vi "Network - Send Start Session.vi"(8 "error in":errorcluster, 9 "Info":string, 10 "URL":string="127.0.0.1", 11 "Numeric":dbl) -> (0 "error out":errorcluster)   [LabVIEW 2010, in "Core SubVIs.lvlib"]
uses:
  Core SubVIs.lvlib
panel:
  out "Connected":bool
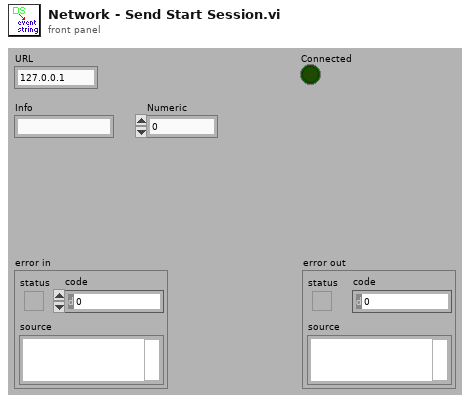
[diagram p1: front panel]
types:
  T1 = enum16{"Read", "Write", "ReadWrite", "BufferedRead", "BufferedReadWrite"}
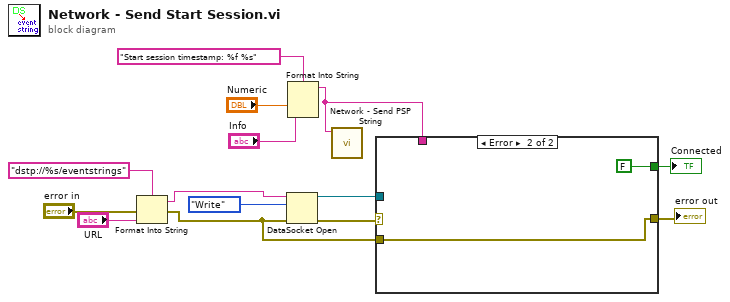
[diagram p0: block diagram]
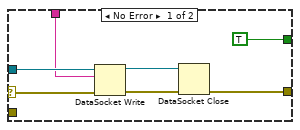
[diagram p2: hidden frame]
diagram:
  n1 = Format Into String(format string="dstp://%s/eventstrings", error in="error in", "URL") -> (resulting string=w10:string, error out=w2:errorcluster)  [unwired: 1 in]
  n2 = DataSocket Open(8:w2, 10:T1."Write" ("mode"), 11:w10) -> (0:w8:errorcluster, 3:w14:refnum<k13>)  [unwired: 1 out]
  n3 = Format Into String(format string="Start session timestamp: %f %s", "Numeric", "Info") -> (resulting string=w1:string)  [unwired: 2 in, 1 out]
  n4 = call "Network - Send PSP String.vi"("Message"=w1) -> ()  [unwired: 11 in]
  n5 = case shown="Error" w8 {
    selector: w8 -> [w18 _]
    tunnel: w14 -> [w21 _]
    tunnel: [w17 w22] -> w7
    tunnel: [TRUE FALSE] -> w6
    tunnel: w1 -> [w15 _]
    tunnel: w2 -> [_ w22]
    frame No Error {
      n6 = DataSocket Write(8:w18, 10:w15, 11:w21) -> (0:w20:errorcluster, 3:w19:refnum<k13>)  [unwired: 2 out]
      n7 = DataSocket Close(8:w20, 11:w19) -> (0:w17:errorcluster)  [unwired: 2 out]
    }
    frame Error {
    }
  }
  "error out" <- w7
  "Connected" <- w6
